vi "2x 4wire, 1x 5wire xVDTs + 1 resolver.vi"() -> ()   [LabVIEW 2010]
uses:
  <vilib>/Platform/TimedLoop/XDataNode/XDataNode.xnode
  <vilib>/Platform/TimedLoop/XDataNode/timing_clust.ctl
  <vilib>/Platform/TimedLoop/XDataNode/nitl_modes.ctl
  <vilib>/Platform/TimedLoop/XDataNode/wakeup.ctl
  <vilib>/Platform/TimedLoop/XDataNode/XDNodeRunTimeDep.lvlib
  <vilib>/NI Veristand/FPGA/NI_VS FPGA Support.lvlib
  <userlib>/_NI VeriStand FPGA Support/NI VeriStand FPGA Clock Support/NI_VS FPGA Clock Support.lvlib
panel:
  in  "Resolver0.ScaleFactor1":i32
  in  "Resolver0.ScaleFactor2":i32
  in  "Resolver0.Scale1":fxp<+/-,19,5>
  in  "Resolver0.Scale2":fxp<+/-,19,5>
  in  "xVDT2.ScaleFactor1":i32
  in  "xVDT2.ScaleFactor2":i32
  in  "xVDT2.Scale2":fxp<+/-,19,5>
  in  "xVDT2.Scale1":fxp<+/-,19,5>
  in  "xVDT1.ScaleFactor1":i32
  in  "xVDT1.Scale1":fxp<+/-,19,5>
  in  "xVDT0.ScaleFactor1":i32
  in  "xVDT0.Scale1":fxp<+/-,19,5>
  in  "Generate IRQ":bool
  in  "Use External Timing":bool
  in  "Write to  RTSI":bool
  in  "Loop Rate (usec)":u32
  in  "Start":bool
  # "4 Wire"
  # "4 Wire"
  # "5 Wire"
  # "Resolver"
  # "Configuration"
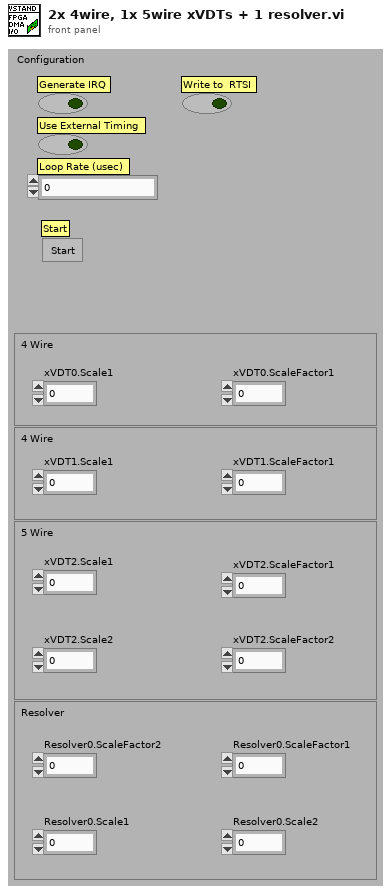
[diagram p1: front panel]
types:
  T1 = typedef "XDNodeRunTimeDep.lvlib/timing_clust.ctl" = cluster{"Expected End [f-1]":u64, "Actual End [f-1]":u64, "Finished Late? [f-1]":bool, "Expected End [i-1]":u64, "Actual End [i-1]":u64, "Finished Late? [i-1]":bool, "Expected Start [i]":u64, "Actual Start [i]":u64, "Expected Start [f]":u64, "Actual Start [f]":u64, "Source Name":string, "Structure Name":string, "Period":i64, "Deadline":i64, "Offset":i64, "Start":i64, "Priority":i32, "Timeout":i32, "Mode":T2, "Wakeup Reason":T3, "Error":errorcluster, "Source Type":string, "Secondary Source Type":string, "Global End Time":u64, "Global Start Time":u64, "Frame Duration":u64, "Iteration Duration":u64, "Assigned CPU":i32, "I/O Scan Engine Mode":u32}
  T2 = typedef "XDNodeRunTimeDep.lvlib/nitl_modes.ctl" = enum32{"No Change", "Process missed periods, maintain original phase", "Discard missed periods, maintain original phase", "Process missed periods, ignore original phase", "Discard missed periods, ignore original phase"}
  T3 = typedef "XDNodeRunTimeDep.lvlib/wakeup.ctl" = enum32{"Normal", "Aborted", "Asynchronous wakeup", "Timing source error", "Timed loop error", "Timeout"}
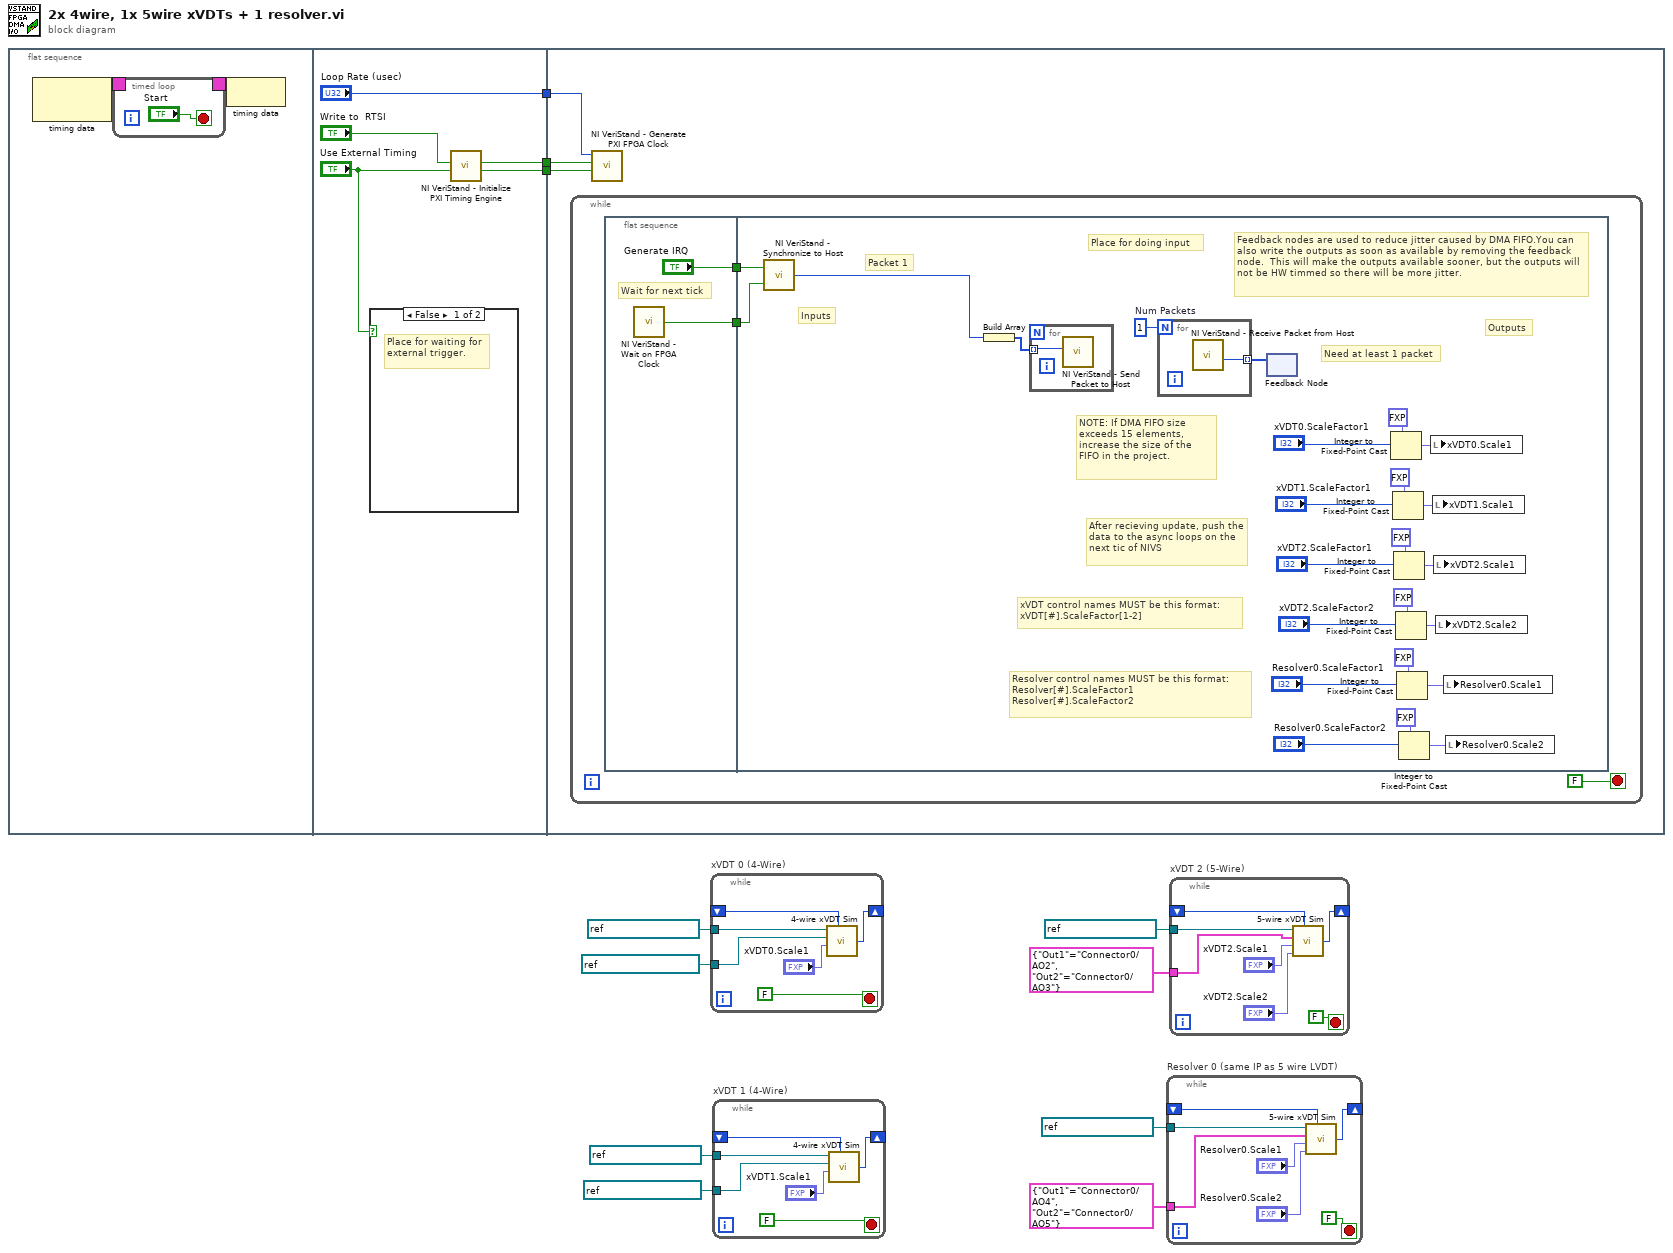
[diagram p0: block diagram]
diagram:
  n1 = flat-sequence {
    tunnel: [w20] -> w11
    tunnel: ["Loop Rate (usec)"] -> w10
    tunnel: [w19] -> w9
    tunnel: w11 -> [w26]
    tunnel: w10 -> [w25]
    tunnel: w9 -> [w24]
    frame #0 {
      n2 = node-c288() -> (w13:T1)  [unwired: 1 out]
      n3 = timed-loop {
        timing: w13 -> [_]
        timing-out: [_] -> w12
        stop <- "Start" stop-if-true
      }
      n4 = node-c288(w12) -> ()
    }
    frame #1 {
      n5 = case shown="False" "Use External Timing" {
        frame False {
          # "Place for waiting for external trigger."
        }
        frame True {
          # "Do not wait on trigger when externally timed."
        }
      }
      n6 = call <userlib>:"NI VeriStand - Initialize PXI Timing Engine.vi"("Use External Timing In"="Use External Timing", "Write to  RTSI In"="Write to  RTSI") -> ("Use External Timing Out"=w20:bool, "Write to  RTSI Out"=w19:bool)  [unwired: 8 in]
    }
    frame #2 {
      n7 = while {
        stop <- FALSE stop-if-true
        n8 = flat-sequence {
          tunnel: ["Generate IRQ"] -> w28
          tunnel: [w30] -> w27
          tunnel: w28 -> [w55]
          tunnel: w27 -> [w54]
          frame #0 {
            # "Wait for next tick"
            n9 = call <userlib>:"NI VeriStand - Wait on FPGA Clock.vi"() -> ("Clock Ticked"=w30:bool)
          }
          frame #1 {
            w51 = 1  # Num Packets
            # "Resolver control names MUST be this format:\nResolver[#].ScaleFactor1\nResolver[#].ScaleFactor2"
            # "xVDT control names MUST be this format:\nxVDT[#].ScaleFactor[1-2]"
            # "After recieving update, push the data to the async loops on the next tic of NIVS"
            # "Need at least 1 packet"
            # "Packet 1"
            # "Inputs"
            # "Outputs"
            # "NOTE: If DMA FIFO size exceeds 15 elements, increase the size of the FIFO in the project."
            # "Feedback nodes are used to reduce jitter caused by DMA FIFO.You can also write the outputs as soon as available by removing the feedback node.  This will make the outputs available sooner, but the outputs will not be HW timmed so there will be more jitter."
            # "Place for doing input"
            n10 = call <userlib>:"NI VeriStand - Synchronize to Host.vi"("Clock Ticked"=w54, "Generate IRQ"=w55) -> ("Is Late?"=w53:u64)
            n11 = Build Array(w53) -> (w52:u64[])
            n12 = for {
              tunnel: w52 -> [w57] mode=indexing
              n13 = call <vilib>:"NI VeriStand - Send Packet to Host.vi"("Element"=w57) -> ()  [unwired: 2 in, 9 out]
            }
            n14 = for {
              N: w51 -> [_]
              tunnel: [w56] -> w50 mode=indexing
              n15 = call <vilib>:"NI VeriStand - Receive Packet from Host.vi"() -> ("Element"=w56:u64)  [unwired: 2 in, 9 out]
            }
            n16 = feedback #1() -> ()  [unwired: 2 in]
            n17 = feedback-in #1(w50) -> ()
            n18 = Integer to Fixed-Point Cast(fixed-point type=fxp<+/-,19,5> 0.0, integer="xVDT0.ScaleFactor1") -> (fixed-point=w48:fxp<+/-,19,5>)
            n19 = Integer to Fixed-Point Cast(fixed-point type=fxp<+/-,19,5> 0.0, integer="xVDT1.ScaleFactor1") -> (fixed-point=w47:fxp<+/-,19,5>)
            n20 = Integer to Fixed-Point Cast(fixed-point type=fxp<+/-,19,5> 0.0, integer="xVDT2.ScaleFactor1") -> (fixed-point=w43:fxp<+/-,19,5>)
            n21 = Integer to Fixed-Point Cast(fixed-point type=fxp<+/-,19,5> 0.0, integer="xVDT2.ScaleFactor2") -> (fixed-point=w44:fxp<+/-,19,5>)
            n22 = Integer to Fixed-Point Cast(fixed-point type=fxp<+/-,19,5> 0.0, integer="Resolver0.ScaleFactor1") -> (fixed-point=w34:fxp<+/-,19,5>)
            n23 = Integer to Fixed-Point Cast(fixed-point type=fxp<+/-,19,5> 0.0, integer="Resolver0.ScaleFactor2") -> (fixed-point=w33:fxp<+/-,19,5>)
            n24 = local write "xVDT0.Scale1"(w48) -> ()
            n25 = local write "xVDT1.Scale1"(w47) -> ()
            n26 = local write "xVDT2.Scale1"(w43) -> ()
            n27 = local write "xVDT2.Scale2"(w44) -> ()
            n28 = local write "Resolver0.Scale1"(w34) -> ()
            n29 = local write "Resolver0.Scale2"(w33) -> ()
          }
        }
      }
      n30 = call <userlib>:"NI VeriStand - Generate PXI FPGA Clock.vi"("Use External Timing"=w26, "Write to  RTSI"=w24, "Loop Rate (usec)"=w25) -> ()  [unwired: 9 in]
    }
  }
  n31 = while "xVDT 0 (4-Wire)" {
    shift-right: [w62] -> _
    shift-left: _ -> [w63]
    tunnel: refnum<k21> "Connector0/AI0" ("FPGA I/O In") -> [w60]
    tunnel: refnum<k21> "Connector0/AO0" ("FPGA I/O In") -> [w59]
    stop <- FALSE stop-if-true
    n32 = call "4-wire xVDT Sim.vi"("Input Channel"=w60, "Output Channel"=w59, "xVDT#.Scale1"="xVDT0.Scale1", "Last Value"=w63) -> ("Next Value"=w62:i16)  [unwired: 1 in]
  }
  n33 = while "xVDT 1 (4-Wire)" {
    shift-right: [w68] -> _
    shift-left: _ -> [w69]
    tunnel: refnum<k21> "Connector0/AI1" ("FPGA I/O In") -> [w66]
    tunnel: refnum<k21> "Connector0/AO1" ("FPGA I/O In") -> [w65]
    stop <- FALSE stop-if-true
    n34 = call "4-wire xVDT Sim.vi"("Input Channel"=w66, "Output Channel"=w65, "xVDT#.Scale1"="xVDT1.Scale1", "Last Value"=w69) -> ("Next Value"=w68:i16)  [unwired: 1 in]
  }
  n35 = while "Resolver 0 (same IP as 5 wire LVDT)" {
    shift-right: [w75] -> _
    shift-left: _ -> [w76]
    tunnel: refnum<k21> "Connector0/AI3" ("FPGA I/O In") -> [w73]
    tunnel: cluster{"Out1":refnum<k21>, "Out2":refnum<k21>} {"Out1"="Connector0/AO4", "Out2"="Connector0/AO5"} ("Output Channels") -> [w72]
    stop <- FALSE stop-if-true
    n36 = call "5-wire xVDT Sim.vi"("Input Channel"=w73, "Output Channels"=w72, "xVDT#.Scale1"="Resolver0.Scale1", "xVDT#.Scale2"="Resolver0.Scale2", "Last Value"=w76) -> ("Next Value"=w75:i16)
  }
  n37 = while "xVDT 2 (5-Wire)" {
    shift-right: [w82] -> _
    shift-left: _ -> [w83]
    tunnel: refnum<k21> "Connector0/AI2" ("FPGA I/O In") -> [w80]
    tunnel: cluster{"Out1":refnum<k21>, "Out2":refnum<k21>} {"Out1"="Connector0/AO2", "Out2"="Connector0/AO3"} ("Output Channels") -> [w79]
    stop <- FALSE stop-if-true
    n38 = call "5-wire xVDT Sim.vi"("Input Channel"=w80, "Output Channels"=w79, "xVDT#.Scale1"="xVDT2.Scale1", "xVDT#.Scale2"="xVDT2.Scale2", "Last Value"=w83) -> ("Next Value"=w82:i16)
  }
